vi "math_ua.vi"(0 "x":dbl[](array[numeric]) format="%0.2f") -> (1 "mean(x)":dbl format="%0.2f", 2 "ua(x)":dbl format="%0.2f", 3 "ua(x) [ppm]":dbl format="%0.2f", 4 "std(x)":dbl format="%0.2f")   [LabVIEW 2020, in "varilib.lvlib"]
doc: "Calculates type A uncertainty of vector of numbers."
uses:
  varilib.lvlib
  <vilib>/Analysis/NI_AALBase.lvlib
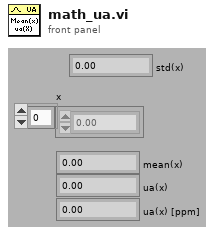
[diagram p1: front panel]
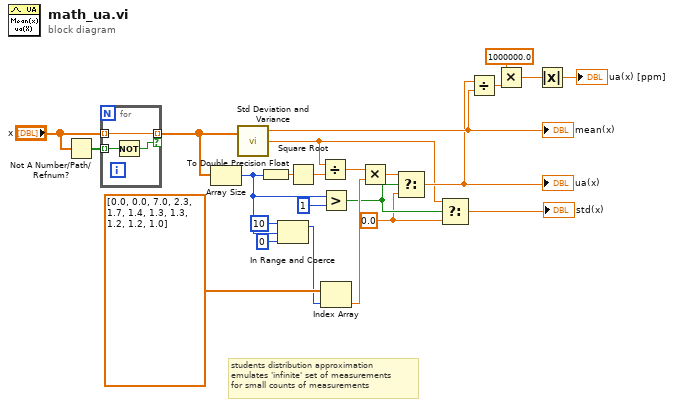
[diagram p0: block diagram]
diagram:
  w4 = 0.0 ("f")
  # "students distribution approximation\nemulates 'infinite' set of measurements\nfor small counts of measurements"
  n1 = Not A Number/Path/Refnum?(number/path/refnum="x") -> (NaN/Path/Refnum?=w3:bool[])
  n2 = for {
    tunnel: w3 -> [w26] mode=indexing
    tunnel: "x" -> [w27] mode=indexing
    tunnel: [w27] -> w1 mode=indexing if=w25
    n3 = Not(x=w26) -> (.not. x?=w25:bool)
  }
  n4 = Array Size(array=w1) -> (size(s)=w11:i32)
  n5 = call <vilib>:"Std Deviation and Variance.vi"("X"=w1) -> ("mean"=w16:dbl, "standard deviation"=w6:dbl)  [unwired: 1 in, 1 out]
  "mean(x)" <- w16
  n6 = To Double Precision Float(number=w11) -> (double precision float=w24:dbl)
  n7 = In Range and Coerce(upper limit=10, x=w11, lower limit=0) -> (coerced(x)=w17:i32)  [unwired: 1 out]
  n8 = Square Root(x=w24) -> (sqrt(x)=w23:dbl)
  n9 = Divide(x=w6, y=w23) -> (x/y=w22:dbl)
  n10 = Greater?(x=w11, y=1) -> (0:w5:bool)
  n11 = Index Array(array=dbl[] [0.0, 0.0, 7.0, 2.3, 1.7, 1.4, 1.3, 1.3, 1.2, 1.2, 1.0], index=w17) -> (element=w18:dbl)
  n12 = Multiply(x=w22, y=w18) -> (x*y=w9:dbl)
  n13 = Select(t=w9, s=w5, f=w4) -> (s? t:f=w8:dbl)
  "ua(x)" <- w8
  n14 = Select(t=w6, s=w5, f=w4) -> (s? t:f=→"std(x)":dbl)
  n15 = Divide(x=w8, y=w16) -> (x/y=w15:dbl)
  n16 = Multiply(x=1000000.0, y=w15) -> (x*y=w12:dbl)
  n17 = Absolute Value(x=w12) -> (abs(x)=→"ua(x) [ppm]":dbl)
